vi "Hab Lifter TeleOp.vi"(11 "Controller Values":T1) -> ()   [LabVIEW 2018]
uses:
  Support Code/Controller Values.ctl
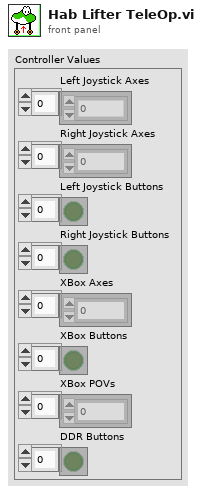
[diagram p1: front panel]
types:
  T1 = typedef "Controller Values.ctl" = cluster{"Left Joystick Axes ":dbl[], "Right Joystick Axes":dbl[], "Left Joystick Buttons":bool[], "Right Joystick Buttons":bool[], "XBox Axes":dbl[], "XBox Buttons":bool[], "XBox POVs":i16[], "DDR Buttons":bool[]}
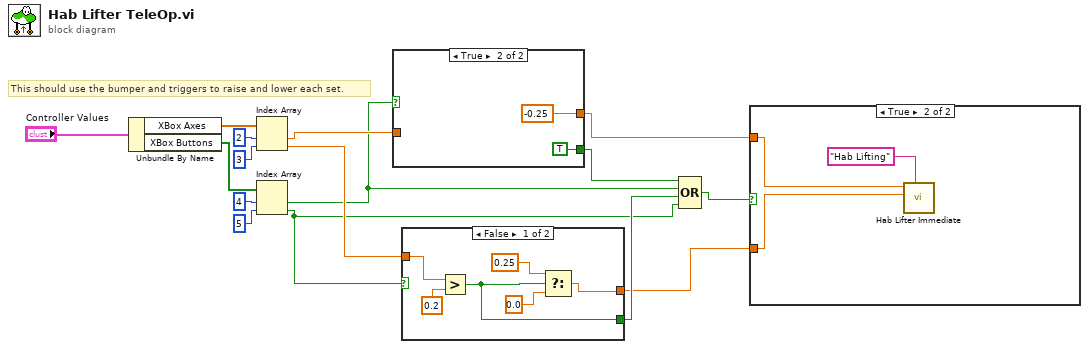
[diagram p0: block diagram]
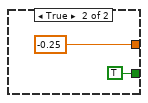
[diagram p3: hidden frame]
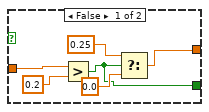
[diagram p4: hidden frame]
diagram:
  # "This should use the bumper and triggers to raise and lower each set."
  n1 = Unbundle By Name("Controller Values") -> ("XBox Axes"=w15:dbl[], "XBox Buttons"=w14:bool[])
  n2 = Index Array(array=w15, index #1=2 ("index"), index #2=3 ("index")) -> (element #1=w9:dbl, element #2=w8:dbl)
  n3 = Index Array(array=w14, index #1=4 ("index"), index #2=5 ("index")) -> (element #1=w6:bool, element #2=w4:bool)
  n4 = case shown="True" w6 {
    tunnel: w9 -> [w22 _]
    tunnel: [w18 -0.25] -> w2
    tunnel: [w17 TRUE] -> w7
    frame False {
      n5 = Greater?(x=w22, y=0.2) -> (0:w17:bool)
      n6 = Select(t=0.25, s=w17, f=0.0) -> (s? t:f=w18:dbl)
    }
    frame True {
    }
  }
  n7 = case shown="False" w4 {
    tunnel: [w26 -0.25] -> w1
    tunnel: w8 -> [w27 _]
    tunnel: [w25 TRUE] -> w5
    frame False {
      n8 = Greater?(x=w27, y=0.2) -> (0:w25:bool)
      n9 = Select(t=0.25, s=w25, f=0.0) -> (s? t:f=w26:dbl)
    }
    frame True {
    }
  }
  n10 = Compound Arithmetic op=OR(w7, w6, w5, w4) -> (w3:bool)
  n11 = case shown="True" w3 {
    tunnel: w2 -> [_ w35]
    tunnel: w1 -> [_ w34]
    frame False {
    }
    frame True {
      n12 = call "Hab Lifter Immediate.vi"("Description"="Hab Lifting", "Right Setpoint"=w34, "Left Setpoint"=w35) -> ()  [unwired: 8 in, 1 out]
    }
  }
